vi "MAIN_STANDALONE.vi"() -> ()   [LabVIEW 2019]
uses:
  Typedefs/ESTADOS.ctl
  Typedefs/Tipo_movimiento.ctl
  Typedefs/Distancia.ctl
  Typedefs/Distancia_Z.ctl
  Typedefs/Cluster_refs_controles.ctl
  Typedefs/Cluster_tracking.ctl
  SHARED TYPES/Acciones_UI.ctl
  Typedefs/Estados_arduino.ctl
  Typedefs/Comandos.ctl
  <vilib>/Instr/_visa.llb/VISA Configure Serial Port (Instr).vi
  <vilib>/Utility/error.llb/Error Cluster From Error Code.vi
  <vilib>/ErrorRing/Error Ring.xnode
  SHARED VI'S/SHARED VI'S.lvlib
  SHARED TYPES/SHARED TYPES.lvlib
panel:
  out "?":u32
  in  "TabDepuracion":enum32{"Page 1", "Page 2"}(tab)
  in  "Tab Control":enum32{"Page 1"}(tab)
  out "Tracking_Z":i32
  in  "Distancia Z":T1=32000 items=["2cm"=64000, "1cm"=32000, "1mm"=3200, "0.5mm"=1600]
  out "Movimiento ejecutado?":bool caption="MOVIMIENTO NO EJECUTADO"
  out "Tracking_Y":i32
  out "Tracking_X":i32
  out "TRAMA DE MOVIMIENTO ENVIADA":string
  out "MENSAJES AL USUARIO":string
  in  "COMENZAR MOVIMIENTO":bool
  in  "HOME":bool
  in  "Avance":bool
  in  "Retroceso":bool
  in  "Derecha":bool
  in  "Izquierda":bool
  in  "STOP PROGRAM":bool
  in  "Sube Z":bool
  in  "Baja Z":bool
  out "ESTADO FSM":T2
  out "MOVIMIENTO SOLICITADO":T3=enum."AVANZAR"
  in  "Distancia X/Y":T4=9100 items=["60cm"=54600, "50cm"=45500, "45cm"=40950, "40cm"=36400, "35cm"=31850, "30cm"=27300, "25cm"=22750, "20cm"=18200, "15cm"=13650, "10cm"=9100, "5cm"=4550, "1cm"=910, "5mm"=455, "1mm"=91, "0.5mm"=45, "0.1mm"=9, "1 paso "=1]
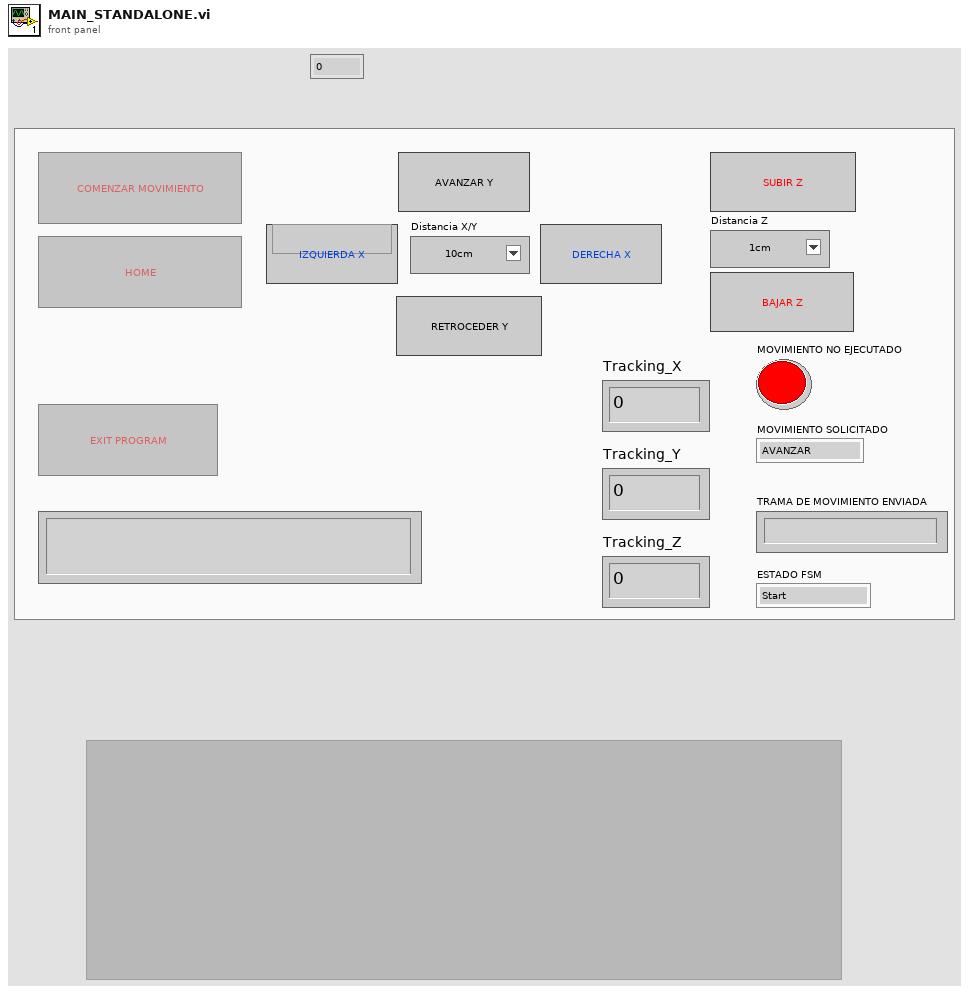
[diagram p1: front panel]
types:
  T1 = typedef "Distancia_Z.ctl" = i32
  T2 = typedef "ESTADOS.ctl" = enum16{"Start", "Ping_Arduino", "Init Refs", "Check Button", "Check Limits", "Home", "Cabezal Posicion Inicio", "Terminaste posicion inicio?", "Terminar", "Salir Arduino", "Envio Parametros Movimiento", "Recepcion Comando?", "Terminaste Movimiento?", "Adquirir Coordenada", "Terminaste Home?", "Salir"}
  T3 = typedef "Tipo_movimiento.ctl" = enum16{"NINGUNO", "AVANZAR", "RETROCEDER", "DERECHA", "IZQUIERDA", "SUBIRZ", "BAJARZ", "HOME", "HOME_Z"}
  T4 = typedef "Distancia.ctl" = i32
  T5 = typedef "Cluster_tracking.ctl" = cluster{"PasosAcumulados_Y":i32, "PasosAcumulados_X":i32, "PasosAcumulados_Z":i32, "Coord.Adquirida_X":i32, "Coord.Adquirida_Y":i32, "Coord.Adquirida_Z":i32}
  T6 = typedef "Cluster_refs_controles.ctl" = cluster{"Comenzar mov":refnum<vi>, "Home":refnum<vi>, "Izq":refnum<vi>, "Der":refnum<vi>, "Stop Program":refnum<vi>, "Avanzar":refnum<vi>, "Bajar Z":refnum<vi>, "Distancia":refnum<vi>, "Subir Z":refnum<vi>, "Retroc":refnum<vi>, "MENSAJES AL USUARIO":refnum<vi>, "Trama enviada":refnum<vi>, "Movimiento ejecutado?":refnum<vi>}
  T7 = typedef "SHARED TYPES.lvlib/Acciones_UI.ctl" = enum16{"Activar", "Desactivar", "Reiniciar default"}
  T8 = enum8{"Enabled", "Disabled", "Disabled and Grayed Out"}
  T9 = typedef "Comandos.ctl" = enum16{"H", "FH", "FI", "FX", "FY", "FZ", "I", "OK"}
  T10 = typedef "Estados_arduino.ctl" = enum16{"2", "3", "4", "5", "6", "7", "9", "8"}
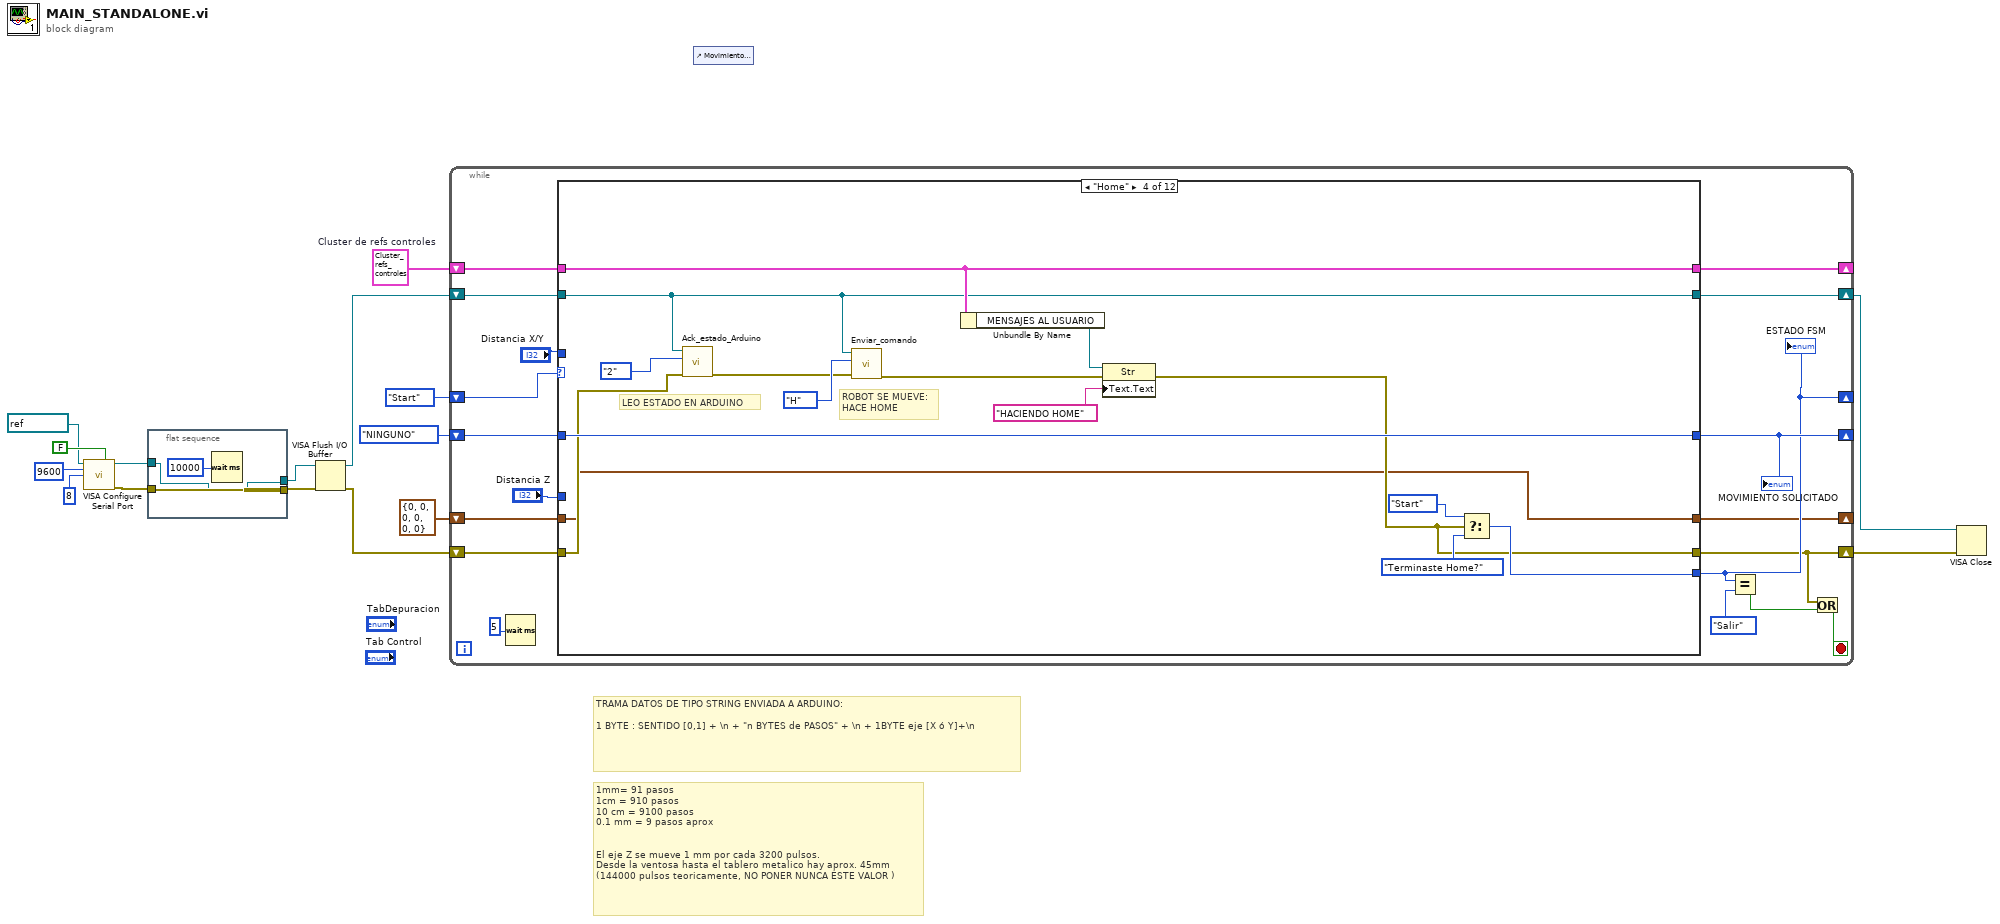
[diagram p0: block diagram]
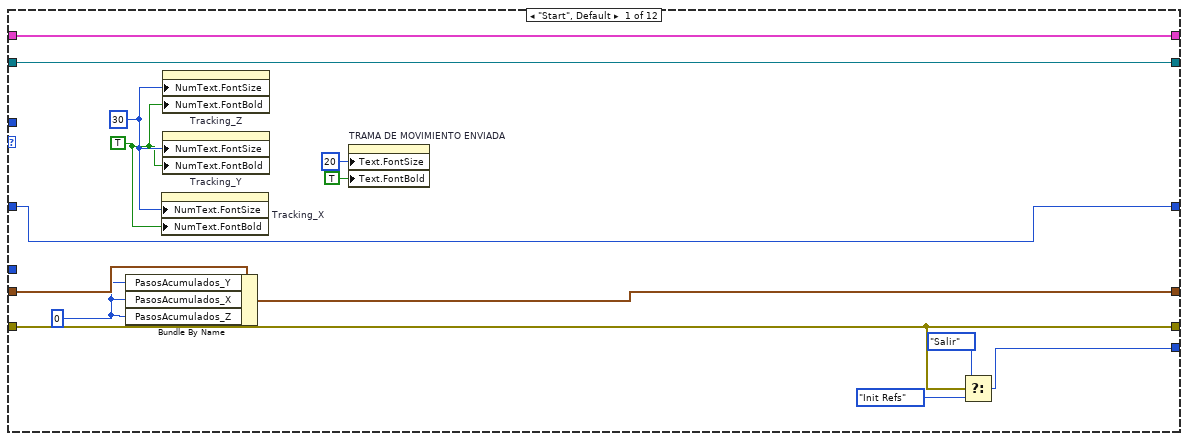
[diagram p2: hidden frame]
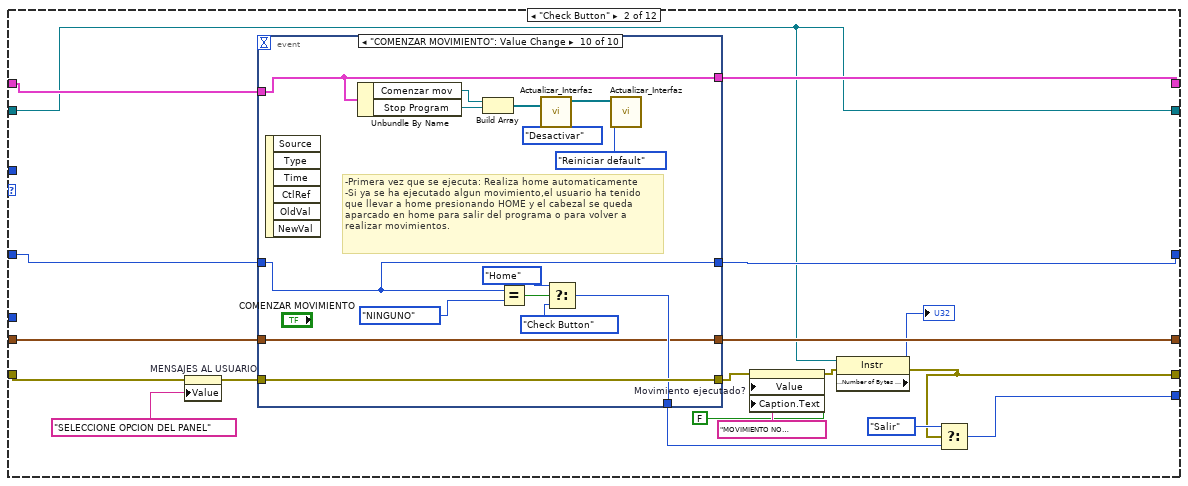
[diagram p3: hidden frame]
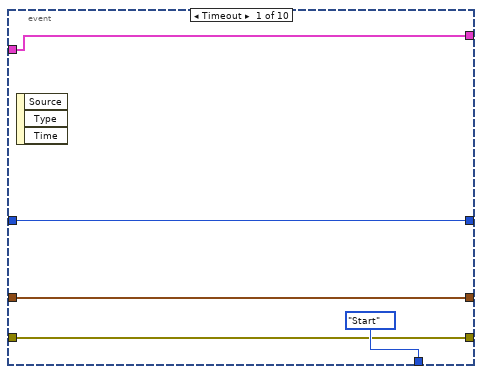
[diagram p4: hidden frame]
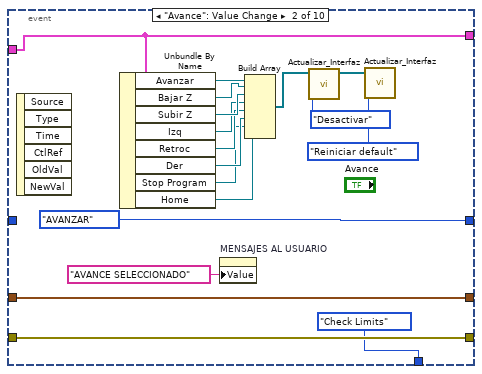
[diagram p5: hidden frame]
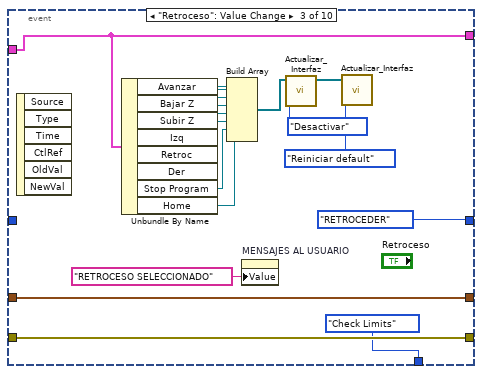
[diagram p6: hidden frame]
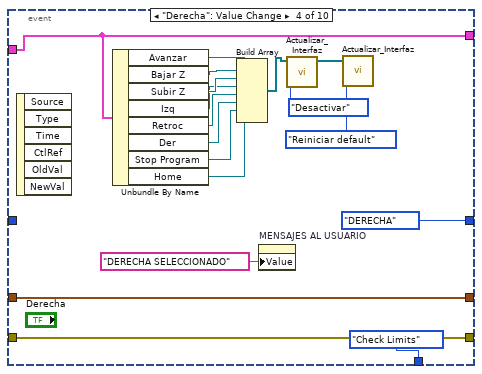
[diagram p7: hidden frame]
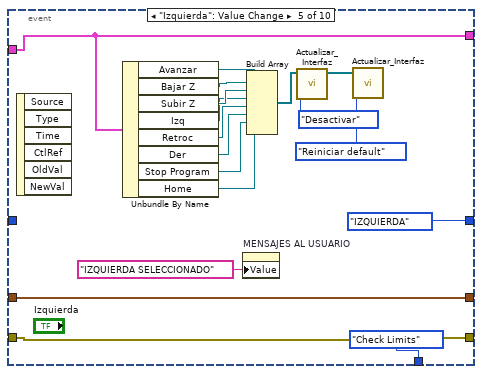
[diagram p8: hidden frame]
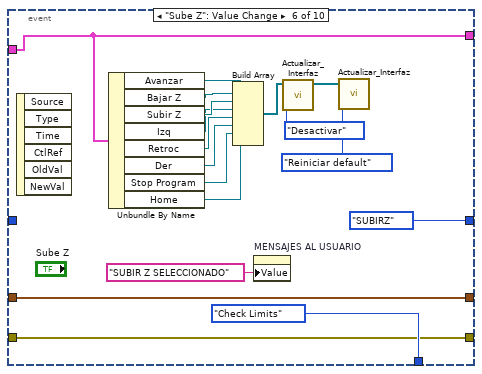
[diagram p9: hidden frame]
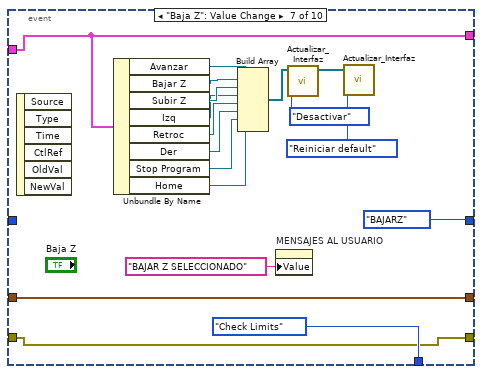
[diagram p10: hidden frame]
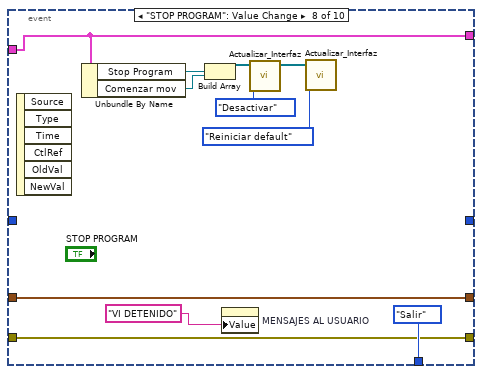
[diagram p11: hidden frame]
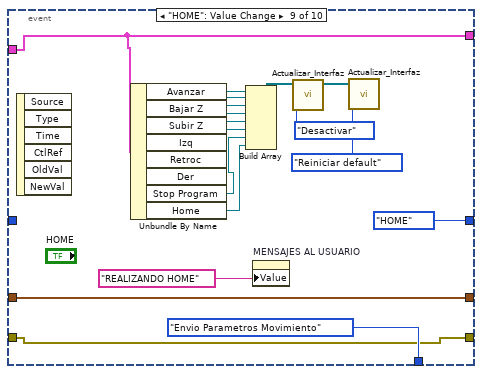
[diagram p12: hidden frame]
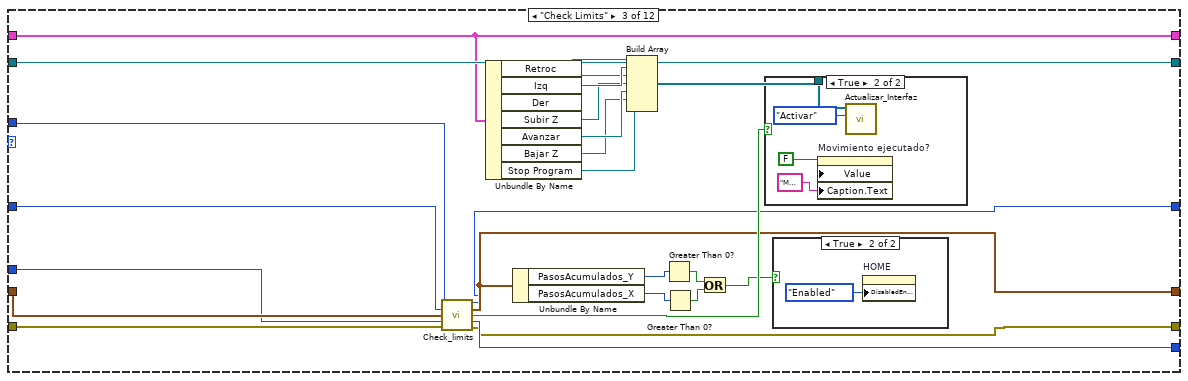
[diagram p13: hidden frame]
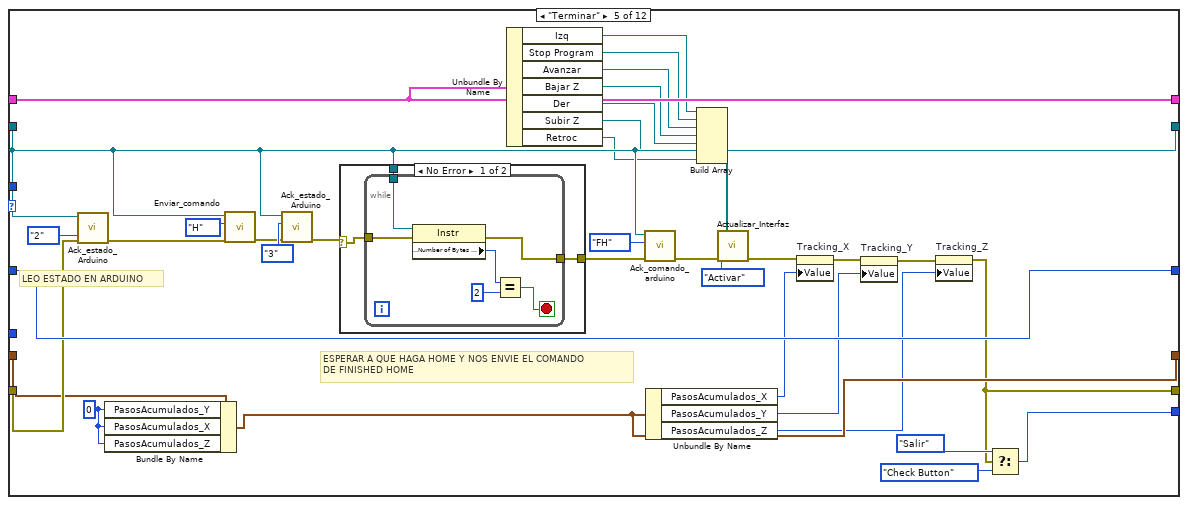
[diagram p16: hidden frame]
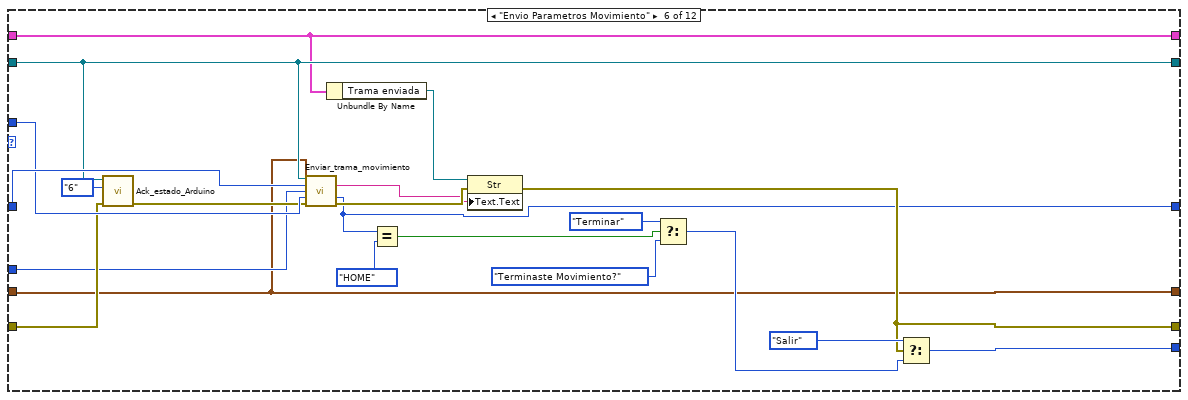
[diagram p18: hidden frame]
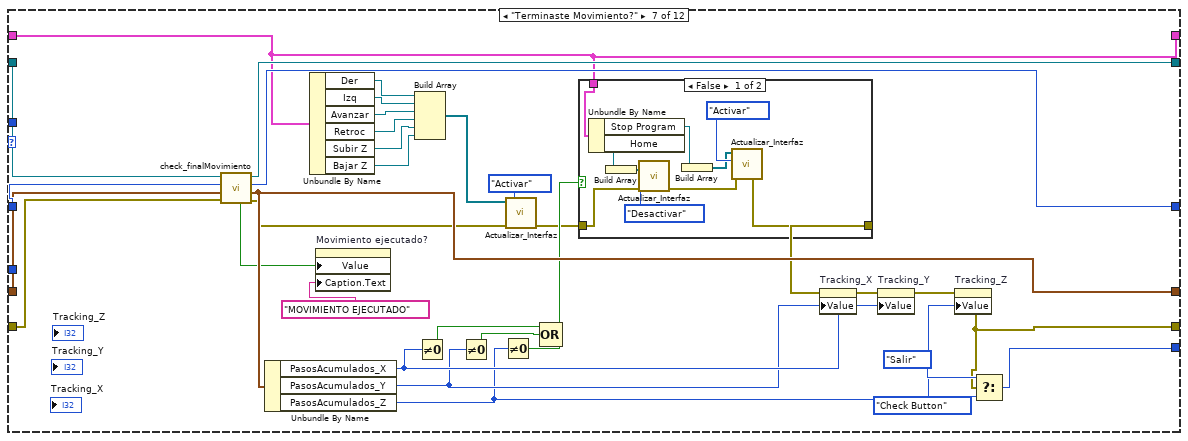
[diagram p19: hidden frame]
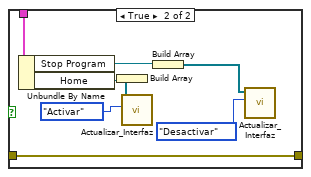
[diagram p20: hidden frame]
diagram:
  w6 = T6 {"Comenzar mov"=refnum, "Home"=refnum, "Izq"=refnum, "Der"=refnum, "Stop Program"=refnum, "Avanzar"=refnum, "Bajar Z"=refnum, "Distancia"=refnum, "Subir Z"=refnum, "Retroc"=refnum, "MENSAJES AL USUARIO"=refnum, "Trama enviada"=refnum, "Movimiento ejecutado?"=refnum}  # Cluster de refs controles
  # "1mm= 91 pasos\n1cm = 910 pasos\n10 cm = 9100 pasos\n0.1 mm = 9 pasos aprox\n\n\nEl eje Z se mueve 1 mm por cada 3200 pulsos. \nDesde la ventosa hasta el tablero metalico hay aprox. 45mm \n(144000 pulsos teoricamente, NO PONER NUNCA ÉSTE VALOR )"
  # "TRAMA DATOS DE TIPO STRING ENVIADA A ARDUINO:\n\n1 BYTE : SENTIDO [0,1] + \\n + \"n BYTES de PASOS\" + \\n + 1BYTE eje [X ó Y]+\\n"
  n1 = call-poly "VISA Configure Serial Port"("VISA resource name"=refnum<visa-resource-name> "COM4", "Enable Termination\nChar (T)"=FALSE ("Enable Termination\nChar (T)"), "baud rate (9600)"=u32 9600, "data bits (8)"=u16 8) -> ("VISA resource name out"=w5:refnum<visa-resource-name>, "error out"=w14:errorcluster)  [unwired: 10 in]
  n2 = flat-sequence {
    tunnel: [w19] -> w9
    tunnel: w14 -> [w19]
    tunnel: [w17] -> w4
    tunnel: w5 -> [w17]
    frame #0 {
      n3 = Wait (ms)(milliseconds to wait=u32 10000) -> ()  [unwired: 1 out]
    }
  }
  n4 = VISA Flush I/O Buffer(VISA resource name=w4, error in (no error)=w9) -> (VISA resource name out=w3:refnum<visa-resource-name>, error out=w2:errorcluster)  [unwired: 1 in]
  n5 = while {
    shift-right: [w25] -> w10
    shift-left: w2 -> [w34]
    shift-right: [w33] -> w11
    shift-left: w3 -> [w35]
    shift-right: [w29] -> _
    shift-left: w6 -> [w30]
    shift-right: [w27] -> _
    shift-left: ESTADOS."Start" ("Enum") -> [w36]
    shift-right: [w31] -> _
    shift-left: Tipo_movimiento."NINGUNO" ("Enum") -> [w32]
    shift-right: [w22] -> _
    shift-left: T5 {"PasosAcumulados_Y"=0, "PasosAcumulados_X"=0, "PasosAcumulados_Z"=0, "Coord.Adquirida_X"=0, "Coord.Adquirida_Y"=0, "Coord.Adquirida_Z"=0} ("Cluster_Tracking") -> [w23]
    stop <- w28 stop-if-true
    n6 = Wait (ms)(milliseconds to wait=u32 5) -> ()  [unwired: 1 out]
    n7 = case shown="\"Home\"" w36 {
      tunnel: w35 -> [w47 w52 w252 w259 w296 w335 w369 w410 w447 w465 w483 w524]
      tunnel: w34 -> [w51 w61 w250 w262 w305 w334 w368 w411 w443 w467 w484 w533]
      tunnel: [w51 w53 w231 w266 w273 w321 w351 w390 w443 w463 w482 w523] -> w25
      tunnel: [w48 w67 w249 w270 w302 w331 w365 w412 w444 w466 w486 w527] -> w27
      tunnel: [w47 w52 w252 w259 w296 w335 w370 w413 w447 w465 w483 w524] -> w33
      tunnel: w32 -> [w46 w64 w248 w271 w307 w338 w371 _ _ _ _ _]
      tunnel: "Distancia X/Y" -> [_ _ w251 _ _ w337 _ _ _ _ _ _]
      tunnel: [w46 w66 w229 w271 w307 w320 w364 _ _ _ _ _] -> w31
      tunnel: w30 -> [w42 w70 w247 w267 w293 w325 w347 w405 w461 w464 w485 w526]
      tunnel: [w42 w69 w247 w267 w293 w325 w347 w405 w448 w464 w485 w526] -> w29
      tunnel: w23 -> [w45 w63 w238 w261 w287 w318 w361 w406 w438 w462 w481 w525]
      tunnel: [w44 w62 w233 w261 w284 w318 w360 w406 w438 w462 w481 w525] -> w22
      tunnel: "Distancia Z" -> [_ _ w230 _ _ w319 _ _ _ _ _ _]
      frame "Start", Default {
        w41 = u32 30 ("Text.Font:Size")
        w40 = TRUE ("Text.Font:Bold")
        w43 = 0 ("PasosAcumulados_Y")
        n8 = Bundle By Name(cluster=w45, "PasosAcumulados_Y"=w43, "PasosAcumulados_X"=w43, "PasosAcumulados_Z"=w43) -> (w44:T5)
        n9 = property on="Tracking_X" class="DigNum (strict)"("NumText.FontSize"=w41, "NumText.FontBold"=w40) -> ()  [unwired: 2 in, 2 out]
        n10 = property on="Tracking_Z" class="DigNum (strict)"("NumText.FontSize"=w41, "NumText.FontBold"=w40) -> ()  [unwired: 2 in, 2 out]
        n11 = property on="Tracking_Y" class="DigNum (strict)"("NumText.FontSize"=w41, "NumText.FontBold"=w40) -> ()  [unwired: 2 in, 2 out]
        n12 = property on="TRAMA DE MOVIMIENTO ENVIADA" class="Str"("Text.FontSize"=u32 20 ("Text.Font:Size"), "Text.FontBold"=TRUE ("Text.Font:Bold")) -> ()  [unwired: 2 in, 2 out]
        n13 = Select(t=ESTADOS."Salir", s=w51, f=ESTADOS."Init Refs" ("Enum")) -> (s? t:f=w48:T2)
      }
      frame "Check Button" {
        n14 = property on="MENSAJES AL USUARIO" class="Str"(error in=w61, "Value"="SELECCIONE OPCION DEL PANEL" ("MENSAJES AL USUARIO")) -> (error out=w60:errorcluster)  [unwired: 1 in, 1 out]
        n15 = event shown="[9] \"COMENZAR MOVIMIENTO\": Value Change" {
          selector: _ -> [_ _ _ _ _ _ _ _ _ _]
          dyn-events: _ -> [_ _ _ _ _ _ _ _ _ _]
          timeout: _ -> [_ _ _ _ _ _ _ _ _ _]
          tunnel: w70 -> [w75 w93 w102 w120 w136 w152 w170 w189 w199 w224]
          tunnel: [w75 w93 w102 w120 w136 w152 w170 w189 w199 w224] -> w69
          tunnel: [w74 Tipo_movimiento."AVANZAR" Tipo_movimiento."RETROCEDER" Tipo_movimiento."DERECHA" Tipo_movimiento."IZQUIERDA" Tipo_movimiento."SUBIRZ" Tipo_movimiento."BAJARZ" _ Tipo_movimiento."HOME" w216] -> w66
          tunnel: [ESTADOS."Start" ESTADOS."Check Limits" ("f") ESTADOS."Check Limits" ("f") ESTADOS."Check Limits" ("f") ESTADOS."Check Limits" ("f") ESTADOS."Check Limits" ("Enum") ESTADOS."Check Limits" ("Enum") ESTADOS."Salir" ("Enum") ESTADOS."Envio Parametros Movimiento" w215] -> w65
          tunnel: [w72 w79 w96 w114 w132 w163 w181 w187 w211 w221] -> w56
          tunnel: w60 -> [w72 w79 w96 w114 w132 w163 w181 w187 w211 w221]
          tunnel: w64 -> [w74 _ _ _ _ _ _ _ _ w216]
          tunnel: w63 -> [w71 w78 w97 w115 w133 w149 w167 w186 w196 w213]
          tunnel: [w71 w78 w97 w115 w133 w149 w167 w186 w196 w213] -> w62
          event Timeout {
            n16 = event-data() -> ()  [unwired: 1 in, 3 out]
          }
          event "Avance": Value Change {
            n17 = event-data() -> ()  [unwired: 1 in, 6 out]
            n18 = Unbundle By Name(w93) -> ("Avanzar"=w92:refnum<vi>, "Bajar Z"=w87:refnum<vi>, "Subir Z"=w86:refnum<vi>, "Izq"=w85:refnum<vi>, "Retroc"=w84:refnum<vi>, "Der"=w83:refnum<vi>, "Stop Program"=w82:refnum<vi>, "Home"=w81:refnum<vi>)
            n19 = property on="MENSAJES AL USUARIO" class="Str"("Value"="AVANCE SELECCIONADO" ("MENSAJES AL USUARIO")) -> ()  [unwired: 2 in, 2 out]
            n20 = Build Array(w92, w87, w86, w85, w84, w83, w82, w81) -> (w91:refnum<vi>[])
            n21 = call "Actualizar_Interfaz.vi"("Enum"=Acciones_UI."Desactivar", "Controls"=w91) -> ("Controls 2"=w89:refnum<vi>[])  [unwired: 8 in, 1 out]
            n22 = call "Actualizar_Interfaz.vi"("Enum"=Acciones_UI."Reiniciar default", "Controls"=w89) -> ()  [unwired: 8 in, 2 out]
          }
          event "Retroceso": Value Change {
            n23 = event-data() -> ()  [unwired: 1 in, 6 out]
            n24 = Unbundle By Name(w102) -> ("Avanzar"=w111:refnum<vi>, "Bajar Z"=w107:refnum<vi>, "Subir Z"=w106:refnum<vi>, "Izq"=w105:refnum<vi>, "Retroc"=w104:refnum<vi>, "Der"=w103:refnum<vi>, "Stop Program"=w100:refnum<vi>, "Home"=w99:refnum<vi>)
            n25 = Build Array(w111, w107, w106, w105, w104, w103, w100, w99) -> (w101:refnum<vi>[])
            n26 = property on="MENSAJES AL USUARIO" class="Str"("Value"="RETROCESO SELECCIONADO" ("MENSAJES AL USUARIO")) -> ()  [unwired: 2 in, 2 out]
            n27 = call "Actualizar_Interfaz.vi"("Enum"=Acciones_UI."Desactivar", "Controls"=w101) -> ("Controls 2"=w109:refnum<vi>[])  [unwired: 8 in, 1 out]
            n28 = call "Actualizar_Interfaz.vi"("Enum"=Acciones_UI."Reiniciar default", "Controls"=w109) -> ()  [unwired: 8 in, 2 out]
          }
          event "Derecha": Value Change {
            n29 = event-data() -> ()  [unwired: 1 in, 6 out]
            n30 = Unbundle By Name(w120) -> ("Avanzar"=w129:refnum<vi>, "Bajar Z"=w125:refnum<vi>, "Subir Z"=w124:refnum<vi>, "Izq"=w123:refnum<vi>, "Retroc"=w122:refnum<vi>, "Der"=w121:refnum<vi>, "Stop Program"=w119:refnum<vi>, "Home"=w117:refnum<vi>)
            n31 = Build Array(w129, w125, w124, w123, w122, w121, w119, w117) -> (w118:refnum<vi>[])
            n32 = property on="MENSAJES AL USUARIO" class="Str"("Value"="DERECHA SELECCIONADO" ("MENSAJES AL USUARIO")) -> ()  [unwired: 2 in, 2 out]
            n33 = call "Actualizar_Interfaz.vi"("Enum"=Acciones_UI."Desactivar", "Controls"=w118) -> ("Controls 2"=w127:refnum<vi>[])  [unwired: 8 in, 1 out]
            n34 = call "Actualizar_Interfaz.vi"("Enum"=Acciones_UI."Reiniciar default", "Controls"=w127) -> ()  [unwired: 8 in, 2 out]
          }
          event "Izquierda": Value Change {
            n35 = event-data() -> ()  [unwired: 1 in, 6 out]
            n36 = Unbundle By Name(w136) -> ("Avanzar"=w147:refnum<vi>, "Bajar Z"=w143:refnum<vi>, "Subir Z"=w142:refnum<vi>, "Izq"=w141:refnum<vi>, "Retroc"=w140:refnum<vi>, "Der"=w139:refnum<vi>, "Stop Program"=w138:refnum<vi>, "Home"=w135:refnum<vi>)
            n37 = property on="MENSAJES AL USUARIO" class="Str"("Value"="IZQUIERDA SELECCIONADO" ("MENSAJES AL USUARIO")) -> ()  [unwired: 2 in, 2 out]
            n38 = Build Array(w147, w143, w142, w141, w140, w139, w138, w135) -> (w137:refnum<vi>[])
            n39 = call "Actualizar_Interfaz.vi"("Enum"=Acciones_UI."Desactivar", "Controls"=w137) -> ("Controls 2"=w145:refnum<vi>[])  [unwired: 8 in, 1 out]
            n40 = call "Actualizar_Interfaz.vi"("Enum"=Acciones_UI."Reiniciar default", "Controls"=w145) -> ()  [unwired: 8 in, 2 out]
          }
          event "Sube Z": Value Change {
            n41 = event-data() -> ()  [unwired: 1 in, 6 out]
            n42 = Unbundle By Name(w152) -> ("Avanzar"=w162:refnum<vi>, "Bajar Z"=w158:refnum<vi>, "Subir Z"=w157:refnum<vi>, "Izq"=w156:refnum<vi>, "Retroc"=w155:refnum<vi>, "Der"=w154:refnum<vi>, "Stop Program"=w153:refnum<vi>, "Home"=w150:refnum<vi>)
            n43 = Build Array(w162, w158, w157, w156, w155, w154, w153, w150) -> (w151:refnum<vi>[])
            n44 = property on="MENSAJES AL USUARIO" class="Str"("Value"="SUBIR Z SELECCIONADO" ("MENSAJES AL USUARIO")) -> ()  [unwired: 2 in, 2 out]
            n45 = call "Actualizar_Interfaz.vi"("Enum"=Acciones_UI."Desactivar", "Controls"=w151) -> ("Controls 2"=w160:refnum<vi>[])  [unwired: 8 in, 1 out]
            n46 = call "Actualizar_Interfaz.vi"("Enum"=Acciones_UI."Reiniciar default", "Controls"=w160) -> ()  [unwired: 8 in, 2 out]
          }
          event "Baja Z": Value Change {
            n47 = event-data() -> ()  [unwired: 1 in, 6 out]
            n48 = Unbundle By Name(w170) -> ("Avanzar"=w180:refnum<vi>, "Bajar Z"=w176:refnum<vi>, "Subir Z"=w175:refnum<vi>, "Izq"=w174:refnum<vi>, "Retroc"=w173:refnum<vi>, "Der"=w172:refnum<vi>, "Stop Program"=w171:refnum<vi>, "Home"=w168:refnum<vi>)
            n49 = Build Array(w180, w176, w175, w174, w173, w172, w171, w168) -> (w169:refnum<vi>[])
            n50 = property on="MENSAJES AL USUARIO" class="Str"("Value"="BAJAR Z SELECCIONADO" ("MENSAJES AL USUARIO")) -> ()  [unwired: 2 in, 2 out]
            n51 = call "Actualizar_Interfaz.vi"("Enum"=Acciones_UI."Desactivar", "Controls"=w169) -> ("Controls 2"=w178:refnum<vi>[])  [unwired: 8 in, 1 out]
            n52 = call "Actualizar_Interfaz.vi"("Enum"=Acciones_UI."Reiniciar default", "Controls"=w178) -> ()  [unwired: 8 in, 2 out]
          }
          event "STOP PROGRAM": Value Change {
            n53 = event-data() -> ()  [unwired: 1 in, 6 out]
            n54 = Unbundle By Name(w189) -> ("Stop Program"=w194:refnum<vi>, "Comenzar mov"=w185:refnum<vi>)
            n55 = Build Array(w194, w185) -> (w193:refnum<vi>[])
            n56 = property on="MENSAJES AL USUARIO" class="Str"("Value"="VI DETENIDO" ("MENSAJES AL USUARIO")) -> ()  [unwired: 2 in, 2 out]
            n57 = call "Actualizar_Interfaz.vi"("Enum"=Acciones_UI."Desactivar", "Controls"=w193) -> ("Controls 2"=w191:refnum<vi>[])  [unwired: 8 in, 1 out]
            n58 = call "Actualizar_Interfaz.vi"("Enum"=Acciones_UI."Reiniciar default", "Controls"=w191) -> ()  [unwired: 8 in, 2 out]
          }
          event "HOME": Value Change {
            n59 = event-data() -> ()  [unwired: 1 in, 6 out]
            n60 = Unbundle By Name(w199) -> ("Avanzar"=w209:refnum<vi>, "Bajar Z"=w204:refnum<vi>, "Subir Z"=w203:refnum<vi>, "Izq"=w202:refnum<vi>, "Retroc"=w201:refnum<vi>, "Der"=w200:refnum<vi>, "Stop Program"=w198:refnum<vi>, "Home"=w197:refnum<vi>)
            n61 = Build Array(w209, w204, w203, w202, w201, w200, w198, w197) -> (w208:refnum<vi>[])
            n62 = property on="MENSAJES AL USUARIO" class="Str"("Value"="REALIZANDO HOME" ("MENSAJES AL USUARIO")) -> ()  [unwired: 2 in, 2 out]
            n63 = call "Actualizar_Interfaz.vi"("Enum"=Acciones_UI."Desactivar", "Controls"=w208) -> ("Controls 2"=w206:refnum<vi>[])  [unwired: 8 in, 1 out]
            n64 = call "Actualizar_Interfaz.vi"("Enum"=Acciones_UI."Reiniciar default", "Controls"=w206) -> ()  [unwired: 8 in, 2 out]
          }
          event "COMENZAR MOVIMIENTO": Value Change {
            # "-Primera vez que se ejecuta: Realiza home automaticamente\n-Si ya se ha ejecutado algun movimiento,el usuario ha tenido que llevar a home presionando HOME y el cabezal se queda aparcado en home para salir del programa o para volver a realizar movimientos."
            n65 = event-data() -> ()  [unwired: 1 in, 6 out]
            n66 = Unbundle By Name(w224) -> ("Comenzar mov"=w227:refnum<vi>, "Stop Program"=w214:refnum<vi>)
            n67 = Build Array(w227, w214) -> (w226:refnum<vi>[])
            n68 = Equal?(x=w216, y=Tipo_movimiento."NINGUNO") -> (x = y?=w219:bool)
            n69 = call "Actualizar_Interfaz.vi"("Enum"=Acciones_UI."Desactivar", "Controls"=w226) -> ("Controls 2"=w223:refnum<vi>[])  [unwired: 8 in, 1 out]
            n70 = Select(t=ESTADOS."Home", s=w219, f=ESTADOS."Check Button") -> (s? t:f=w215:T2)
            n71 = call "Actualizar_Interfaz.vi"("Enum"=Acciones_UI."Reiniciar default", "Controls"=w223) -> ()  [unwired: 8 in, 2 out]
          }
        }
        n72 = property on="Movimiento ejecutado?" class="Bool (strict)"(error in=w56, "Value"=FALSE ("Movimiento ejecutado?"), "Caption.Text"="MOVIMIENTO NO EJECUTADO" ("Label.Text")) -> (error out=w54:errorcluster)  [unwired: 1 in, 1 out]
        n73 = property class="Instr"(reference=w52, error in=w54) -> (error out=w53:errorcluster, "Serial Settings:Number of Bytes at Serial Port"=→"?":u32)  [unwired: 1 out]
        n74 = Select(t=ESTADOS."Salir", s=w53, f=w65) -> (s? t:f=w67:T2)
      }
      frame "Check Limits" {
        n75 = call "Check_limits.vi"("Distancia X/Y"=w251, "Tipo Movimiento"=w248, "Cluster_Tracking"=w238, "Distancia Z"=w230, "error in (no error)"=w250) -> ("Tipo Movimiento 2"=w229:T3, "Cluster_Tracking 2"=w233:T5, "Limite sobrepasado?"=w246:bool, "Estado"=w249:T2, "error out"=w231:errorcluster)  [unwired: 6 in]
        n76 = Unbundle By Name(w247) -> ("Retroc"=w245:refnum<vi>, "Izq"=w244:refnum<vi>, "Der"=w243:refnum<vi>, "Subir Z"=w242:refnum<vi>, "Avanzar"=w241:refnum<vi>, "Bajar Z"=w240:refnum<vi>, "Stop Program"=w228:refnum<vi>)
        n77 = Unbundle By Name(w233) -> ("PasosAcumulados_Y"=w236:i32, "PasosAcumulados_X"=w235:i32)
        n78 = Build Array(w245, w244, w243, w242, w241, w240, w228) -> (w239:refnum<vi>[])
        n79 = Greater Than 0?(x=w236) -> (x > 0?=w237:bool)
        n80 = Greater Than 0?(x=w235) -> (x > 0?=w234:bool)
        n81 = Or(x=w237, y=w234) -> (x .or. y?=w232:bool)
        n82 = case shown="True" w246 {
          tunnel: w239 -> [_ w257]
          frame False {
          }
          frame True {
            n83 = property on="Movimiento ejecutado?" class="Bool (strict)"("Value"=FALSE ("Movimiento ejecutado"), "Caption.Text"="MOVIMIENTO NO EJECUTADO" ("Label.Text")) -> ()  [unwired: 2 in, 2 out]
            n84 = call "Actualizar_Interfaz.vi"("Enum"=Acciones_UI."Activar", "Controls"=w257) -> ()  [unwired: 8 in, 2 out]
          }
        }
        n85 = case shown="True" w232 {
          frame False {
          }
          frame True {
            n86 = property on="HOME" class="Bool"("DisabledEnum"=T8."Enabled" ("Disabled")) -> ()  [unwired: 2 in, 2 out]
          }
        }
      }
      frame "Home" {
        # "ROBOT SE MUEVE:\nHACE HOME"
        # "LEO ESTADO EN ARDUINO"
        n87 = call "Ack_estado_Arduino.vi"("error in (no error)"=w262, "Enum"=Estados_arduino."2", "VISA resource name"=w259) -> ("error out"=w258:errorcluster)  [unwired: 6 in, 2 out]
        n88 = call "Enviar_comando.vi"("error in (no error)"=w258, "Enum"=Comandos."H", "VISA resource name"=w259) -> ("error out"=w265:errorcluster)  [unwired: 6 in, 2 out]
        n89 = Unbundle By Name(w267) -> ("MENSAJES AL USUARIO"=w264:refnum<vi>)
        n90 = property class="Str"(reference=w264, error in=w265, "Text.Text"="HACIENDO HOME") -> (error out=w266:errorcluster)  [unwired: 1 out]
        n91 = Select(t=ESTADOS."Start" ("Enum"), s=w266, f=ESTADOS."Terminaste Home?" ("Enum")) -> (s? t:f=w270:T2)
      }
      frame "Terminar" {
        w276 = 0 ("PasosAcumulados_Y")
        # "LEO ESTADO EN ARDUINO"
        # "ESPERAR A QUE HAGA HOME Y NOS ENVIE EL COMANDO\nDE FINISHED HOME"
        n92 = call "Ack_estado_Arduino.vi"("error in (no error)"=w305, "Enum"=Estados_arduino."2", "VISA resource name"=w296) -> ("error out"=w301:errorcluster)  [unwired: 6 in, 2 out]
        n93 = Bundle By Name(cluster=w287, "PasosAcumulados_Y"=w276, "PasosAcumulados_X"=w276, "PasosAcumulados_Z"=w276) -> (w284:T5)
        n94 = call "Enviar_comando.vi"("error in (no error)"=w301, "Enum"=Comandos."H", "VISA resource name"=w296) -> ("error out"=w295:errorcluster)  [unwired: 6 in, 2 out]
        n95 = call "Ack_estado_Arduino.vi"("error in (no error)"=w295, "Enum"=Estados_arduino."3", "VISA resource name"=w296) -> ("error out"=w297:errorcluster)  [unwired: 6 in, 2 out]
        n96 = case shown="No Error" w297 {
          selector: w297 -> [w308 w317]
          tunnel: [w310 w317] -> w299
          tunnel: w296 -> [w309 _]
          frame No Error {
            n97 = while {
              tunnel: [w316] -> w310
              tunnel: w309 -> [w312]
              tunnel: w308 -> [w311]
              stop <- w313 stop-if-true
              n98 = property class="Instr"(reference=w312, error in=w311) -> (error out=w316:errorcluster, "Serial Settings:Number of Bytes at Serial Port"=w315:u32)  [unwired: 1 out]
              n99 = Equal?(x=w315, y=u32 2) -> (x = y?=w313:bool)
            }
          }
          frame Error {
          }
        }
        n100 = Unbundle By Name(w293) -> ("Izq"=w292:refnum<vi>, "Stop Program"=w288:refnum<vi>, "Avanzar"=w281:refnum<vi>, "Bajar Z"=w280:refnum<vi>, "Der"=w279:refnum<vi>, "Subir Z"=w278:refnum<vi>, "Retroc"=w277:refnum<vi>)
        n101 = call "Ack_comando_arduino.vi"("error in (no error)"=w299, 10:Comandos."FH", "VISA resource name"=w296) -> ("error IO"=w291:errorcluster)  [unwired: 6 in, 2 out]
        n102 = Unbundle By Name(w284) -> ("PasosAcumulados_X"=w283:i32, "PasosAcumulados_Y"=w282:i32, "PasosAcumulados_Z"=w274:i32)
        n103 = Build Array(w292, w288, w281, w280, w279, w278, w277) -> (w290:refnum<vi>[])
        n104 = call "Actualizar_Interfaz.vi"("error in (no error)"=w291, "Enum"=Acciones_UI."Activar", "Controls"=w290) -> ("error out"=w286:errorcluster)  [unwired: 7 in, 1 out]
        n105 = property on="Tracking_X" class="DigNum (strict)"(error in=w286, "Value"=w283) -> (error out=w285:errorcluster)  [unwired: 1 in, 1 out]
        n106 = property on="Tracking_Y" class="DigNum (strict)"(error in=w285, "Value"=w282) -> (error out=w275:errorcluster)  [unwired: 1 in, 1 out]
        n107 = property on="Tracking_Z" class="DigNum (strict)"(error in=w275, "Value"=w274) -> (error out=w273:errorcluster)  [unwired: 1 in, 1 out]
        n108 = Select(t=ESTADOS."Salir" ("Enum"), s=w273, f=ESTADOS."Check Button") -> (s? t:f=w302:T2)
      }
      frame "Envio Parametros Movimiento" {
        n109 = call "Ack_estado_Arduino.vi"("error in (no error)"=w334, "Enum"=Estados_arduino."6", "VISA resource name"=w335) -> ("error out"=w333:errorcluster)  [unwired: 6 in, 2 out]
        n110 = call "Enviar_trama_movimiento.vi"("VISA resource name"=w335, "Cluster_Tracking"=w318, "Tipo movimiento"=w338, "Distancia Z"=w319, "Distancia X/Y"=w337, "error in (no error)"=w333) -> ("TRAMA ENVIADA"=w323:string, "Tipo movimiento"=w320:T3, "error out"=w324:errorcluster)  [unwired: 6 in, 1 out]
        n111 = Unbundle By Name(w325) -> ("Trama enviada"=w322:refnum<vi>)
        n112 = Equal?(x=w320, y=Tipo_movimiento."HOME") -> (x = y?=w329:bool)
        n113 = property class="Str"(reference=w322, error in=w324, "Text.Text"=w323) -> (error out=w321:errorcluster)  [unwired: 1 out]
        n114 = Select(t=ESTADOS."Terminar", s=w329, f=ESTADOS."Terminaste Movimiento?") -> (s? t:f=w326:T2)
        n115 = Select(t=ESTADOS."Salir" ("Enum"), s=w321, f=w326) -> (s? t:f=w331:T2)
      }
      frame "Terminaste Movimiento?" {
        n116 = call "check_finalMovimiento.vi"("error in (no error)"=w368, "Cluster_Tracking in"=w361, "Enum in"=w371, "VISA Refnum in"=w369) -> ("error out"=w352:errorcluster, "Cluster_Tracking out"=w360:T5, "Enum out"=w364:T3, "VISA Refnum out"=w370:refnum<visa-resource-name>, "Movimiento realizado?"=w348:bool)  [unwired: 3 in]
        n117 = Unbundle By Name(w360) -> ("PasosAcumulados_X"=w359:i32, "PasosAcumulados_Y"=w358:i32, "PasosAcumulados_Z"=w353:i32)
        n118 = Unbundle By Name(w347) -> ("Der"=w346:refnum<vi>, "Izq"=w345:refnum<vi>, "Avanzar"=w344:refnum<vi>, "Retroc"=w343:refnum<vi>, "Subir Z"=w342:refnum<vi>, "Bajar Z"=w341:refnum<vi>)
        n119 = property on="Movimiento ejecutado?" class="Bool (strict)"("Value"=w348, "Caption.Text"="MOVIMIENTO EJECUTADO" ("Label.Text")) -> ()  [unwired: 2 in, 2 out]
        n120 = Build Array(w346, w345, w344, w343, w342, w341) -> (w340:refnum<vi>[])
        n121 = Not Equal To 0?(x=w359) -> (x != 0?=w357:bool)
        n122 = Not Equal To 0?(x=w358) -> (x != 0?=w356:bool)
        n123 = Not Equal To 0?(x=w353) -> (x != 0?=w355:bool)
        n124 = call "Actualizar_Interfaz.vi"("Enum"=Acciones_UI."Activar", "Controls"=w340) -> ()  [unwired: 8 in, 2 out]
        n125 = Compound Arithmetic op=OR(w357, w356, w355) -> (w354:bool)
        n126 = case shown="False" w354 {
          tunnel: w352 -> [w376 w386]
          tunnel: [w374 w386] -> w350
          tunnel: w347 -> [w373 w385]
          frame False {
            n127 = Unbundle By Name(w373) -> ("Stop Program"=w377:refnum<vi>, "Home"=w381:refnum<vi>)
            n128 = Build Array(w381) -> (w380:refnum<vi>[])
            n129 = call "Actualizar_Interfaz.vi"("error in (no error)"=w376, "Enum"=Acciones_UI."Desactivar", "Controls"=w380) -> ("error out"=w375:errorcluster)  [unwired: 7 in, 1 out]
            n130 = Build Array(w377) -> (w372:refnum<vi>[])
            n131 = call "Actualizar_Interfaz.vi"("error in (no error)"=w375, "Enum"=Acciones_UI."Activar", "Controls"=w372) -> ("error out"=w374:errorcluster)  [unwired: 7 in, 1 out]
          }
          frame True {
            n132 = Unbundle By Name(w385) -> ("Stop Program"=w384:refnum<vi>, "Home"=w389:refnum<vi>)
            n133 = Build Array(w389) -> (w387:refnum<vi>[])
            n134 = call "Actualizar_Interfaz.vi"("Enum"=Acciones_UI."Activar", "Controls"=w387) -> ()  [unwired: 8 in, 2 out]
            n135 = Build Array(w384) -> (w382:refnum<vi>[])
            n136 = call "Actualizar_Interfaz.vi"("Enum"=Acciones_UI."Desactivar", "Controls"=w382) -> ()  [unwired: 8 in, 2 out]
          }
        }
        n137 = property on="Tracking_X" class="DigNum (strict)"(error in=w350, "Value"=w359) -> (error out=w363:errorcluster)  [unwired: 1 in, 1 out]
        n138 = property on="Tracking_Y" class="DigNum (strict)"(error in=w363, "Value"=w358) -> (error out=w362:errorcluster)  [unwired: 1 in, 1 out]
        n139 = property on="Tracking_Z" class="DigNum (strict)"(error in=w362, "Value"=w353) -> (error out=w351:errorcluster)  [unwired: 1 in, 1 out]
        n140 = Select(t=ESTADOS."Salir" ("Enum"), s=w351, f=ESTADOS."Check Button") -> (s? t:f=w365:T2)
      }
      frame "Terminaste Home?" {
        # "LEO ESTADO EN ARDUINO"
        # "ESPERAR A QUE HAGA HOME Y NOS ENVIE EL COMANDO\nDE FINISHED HOME \"FH\""
        n141 = call "Ack_estado_Arduino.vi"("error in (no error)"=w411, "Enum"=Estados_arduino."3", "VISA resource name"=w410) -> ("error out"=w407:errorcluster, "VISA resource name out"=w408:refnum<visa-resource-name>)  [unwired: 6 in, 1 out]
        n142 = case shown="No Error" w407 {
          selector: w407 -> [w419 w430]
          tunnel: [w422 w430] -> w415
          tunnel: [w421 w431] -> w414
          tunnel: w408 -> [w420 w431]
          frame No Error {
            n143 = while {
              tunnel: [w429] -> w422
              tunnel: w420 -> [w426]
              tunnel: [w424] -> w421
              tunnel: w419 -> [w425]
              stop <- w427 stop-if-true
              n144 = property class="Instr"(reference=w426, error in=w425) -> (reference out=w424:refnum<visa-resource-name>, error out=w429:errorcluster, "Serial Settings:Number of Bytes at Serial Port"=w423:u32)
              n145 = Equal?(x=w423, y=u32 2) -> (x = y?=w427:bool)
            }
          }
          frame Error {
          }
        }
        n146 = Unbundle By Name(w405) -> ("Retroc"=w402:refnum<vi>, "Izq"=w401:refnum<vi>, "Der"=w400:refnum<vi>, "Subir Z"=w399:refnum<vi>, "Avanzar"=w398:refnum<vi>, "Bajar Z"=w397:refnum<vi>, "Distancia"=w396:refnum<vi>, "Stop Program"=w395:refnum<vi>, "Movimiento ejecutado?"=w393:refnum<vi>)
        n147 = call "Ack_comando_arduino.vi"("error in (no error)"=w415, 10:Comandos."FH", "VISA resource name"=w414) -> ("error IO"=w404:errorcluster, "VISA resource name 2"=w413:refnum<visa-resource-name>)  [unwired: 6 in, 1 out]
        n148 = Build Array(w402, w401, w400, w399, w398, w397, w396, w395, w393) -> (w394:refnum<vi>[])
        n149 = call "Actualizar_Interfaz.vi"("error in (no error)"=w404, "Enum"=Acciones_UI."Activar", "Controls"=w394) -> ("error out"=w392:errorcluster)  [unwired: 7 in, 1 out]
        n150 = property on="Distancia Z" class="Ring (strict)"(error in=w392, "DisabledEnum"=T8."Enabled" ("Disabled")) -> (error out=w390:errorcluster)  [unwired: 1 in, 1 out]
        n151 = Select(t=ESTADOS."Salir" ("Enum"), s=w390, f=ESTADOS."Check Button") -> (s? t:f=w412:T2)
      }
      frame "Init Refs" {
        n152 = control-ref of="Izquierda"() -> (w457:refnum<vi>)
        n153 = control-ref of="HOME"() -> (w458:refnum<vi>)
        n154 = control-ref of="Derecha"() -> (w456:refnum<vi>)
        n155 = control-ref of="STOP PROGRAM"() -> (w455:refnum<vi>)
        n156 = control-ref of="Avance"() -> (w454:refnum<vi>)
        n157 = control-ref of="COMENZAR MOVIMIENTO"() -> (w442:refnum<vi>)
        n158 = control-ref of="Baja Z"() -> (w453:refnum<vi>)
        n159 = control-ref of="Distancia xy"() -> (w437:refnum<vi>)
        n160 = control-ref of="Sube Z"() -> (w452:refnum<vi>)
        n161 = control-ref of="Retroceso"() -> (w451:refnum<vi>)
        n162 = control-ref of="Movimiento ejecutado?"() -> (w436:refnum<vi>)
        n163 = control-ref of="MENSAJES AL USUARIO"() -> (w434:refnum<vi>)
        n164 = control-ref of="TRAMA DE MOVIMIENTO ENVIADA"() -> (w439:refnum<vi>)
        n165 = property class="Str"(reference=w434, "Text.FontSize"=u32 30 ("Text.Font:Size"), "Text.FontBold"=TRUE ("Text.Font:Bold")) -> ()  [unwired: 1 in, 2 out]
        n166 = Bundle By Name(cluster=w461, "Comenzar mov"=w442, "Home"=w458, "Izq"=w457, "Der"=w456, "Stop Program"=w455, "Avanzar"=w454, "Bajar Z"=w453, "Distancia"=w437, "Subir Z"=w452, "Retroc"=w451, "MENSAJES AL USUARIO"=w434, "Trama enviada"=w439, "Movimiento ejecutado?"=w436) -> (w448:T6)
        n167 = property on="Distancia Z" class="Ring (strict)"("DisabledEnum"=T8."Disabled and Grayed Out" ("Disabled")) -> ()  [unwired: 2 in, 2 out]
        n168 = Build Array(w458, w457, w456, w455, w454, w453, w437, w452, w451, w442, w436) -> (w450:refnum<vi>[])
        n169 = call "Actualizar_Interfaz.vi"("Enum"=Acciones_UI."Desactivar", "Controls"=w450) -> ()  [unwired: 8 in, 2 out]
        n170 = Build Array(w434) -> (w459:refnum<vi>[])
        n171 = call "Actualizar_Interfaz.vi"("Enum"=Acciones_UI."Activar", "Controls"=w459) -> ("Controls 2"=w441:refnum<vi>[])  [unwired: 8 in, 1 out]
        n172 = call "Actualizar_Interfaz.vi"("Enum"=Acciones_UI."Reiniciar default", "Controls"=w441) -> ()  [unwired: 8 in, 2 out]
        n173 = Select(t=ESTADOS."Salir" ("Enum"), s=w443, f=ESTADOS."Ping_Arduino") -> (s? t:f=w444:T2)
      }
      frame "Cabezal Posicion Inicio" {
        n174 = disable-structure shown="Disabled" {
          disable-tunnel: w467 -> [w479 _]
          disable-tunnel: [w475 _] -> w466
          disable-tunnel: w465 -> [w473 _]
          disable-tunnel: w464 -> [w472 _]
          disable-tunnel: [w469 _] -> w463
          frame Disabled {
            # "ENVIO COMANDO PARA POSICION INICIO\nEL ROBOT SE EMPIEZA A MOVER A POSICION\nINICIO"
            # "LEO ESTADO EN ARDUINO"
            n175 = call "Ack_estado_Arduino.vi"("error in (no error)"=w479, "Enum"=Estados_arduino."4", "VISA resource name"=w473) -> ("error out"=w478:errorcluster)  [unwired: 6 in, 2 out]
            n176 = call "Enviar_comando.vi"("error in (no error)"=w478, "Enum"=Comandos."I", "VISA resource name"=w473) -> ("error out"=w470:errorcluster)  [unwired: 6 in, 2 out]
            n177 = Unbundle By Name(w472) -> ("MENSAJES AL USUARIO"=w471:refnum<vi>)
            n178 = property class="Str"(reference=w471, error in=w470, "Text.Text"="CABEZAL YENDO A POSICION DE INICIO") -> (error out=w469:errorcluster)  [unwired: 1 out]
            n179 = Select(t=ESTADOS."Salir", s=w469, f=ESTADOS."Terminaste posicion inicio?" ("Enum")) -> (s? t:f=w475:T2)
          }
          frame Enabled {
          }
        }
      }
      frame "Terminaste posicion inicio?" {
        n180 = disable-structure shown="Disabled" {
          disable-tunnel: [w506 _] -> w486
          disable-tunnel: w485 -> [w505 _]
          disable-tunnel: w484 -> [w493 _]
          disable-tunnel: w483 -> [w492 _]
          disable-tunnel: [w491 _] -> w482
          frame Disabled {
            # "LEO ESTADO EN ARDUINO"
            # "ESPERAR A QUE SE VAYA\nA POSICION INICIO Y NOS ENVIE EL COMANDO\n\"FI\""
            # "ESPERO COMANDO POSICION INICIO\nFINALIZADA"
            n181 = call "Ack_estado_Arduino.vi"("error in (no error)"=w493, "Enum"=Estados_arduino."5", "VISA resource name"=w492) -> ("error out"=w507:errorcluster)  [unwired: 6 in, 2 out]
            n182 = case shown="No Error" w507 {
              selector: w507 -> [w513 w522]
              tunnel: [w515 w522] -> w509
              tunnel: w492 -> [w514 _]
              frame No Error {
                n183 = while {
                  tunnel: [w521] -> w515
                  tunnel: w514 -> [w517]
                  tunnel: w513 -> [w516]
                  stop <- w518 stop-if-true
                  # "POLLING"
                  n184 = property class="Instr"(reference=w517, error in=w516) -> (error out=w521:errorcluster, "Serial Settings:Number of Bytes at Serial Port"=w520:u32)  [unwired: 1 out]
                  n185 = Equal?(x=w520, y=u32 2) -> (x = y?=w518:bool)
                }
              }
              frame Error {
              }
            }
            n186 = call "Ack_comando_arduino.vi"("error in (no error)"=w509, 10:Comandos."FI", "VISA resource name"=w492) -> ("error IO"=w490:errorcluster)  [unwired: 6 in, 2 out]
            n187 = Unbundle By Name(w505) -> ("Retroc"=w504:refnum<vi>, "Home"=w503:refnum<vi>, "Izq"=w502:refnum<vi>, "Der"=w501:refnum<vi>, "Stop Program"=w500:refnum<vi>, "Avanzar"=w499:refnum<vi>, "Bajar Z"=w498:refnum<vi>, "Distancia"=w497:refnum<vi>, "Subir Z"=w496:refnum<vi>, "MENSAJES AL USUARIO"=w489:refnum<vi>)
            n188 = property class="Str"(reference=w489, error in=w490, "Text.Text"="CABEZAL EN POSICION DE INICIO") -> (error out=w487:errorcluster)  [unwired: 1 out]
            n189 = Build Array(w504, w503, w502, w501, w500, w499, w498, w497, w496) -> (w495:refnum<vi>[])
            n190 = call "Actualizar_Interfaz.vi"("error in (no error)"=w487, "Enum"=Acciones_UI."Activar", "Controls"=w495) -> ("error out"=w491:errorcluster)  [unwired: 7 in, 1 out]
            n191 = Select(t=ESTADOS."Salir" ("Enum"), s=w491, f=ESTADOS."Check Button") -> (s? t:f=w506:T2)
          }
          frame Enabled {
          }
        }
      }
      frame "Ping_Arduino" {
        n192 = VISA Write(VISA resource name=w524, write buffer="Q?", error in (no error)=w533) -> (return count=w536:u32, error out=w535:errorcluster)  [unwired: 1 out]
        n193 = VISA Read(VISA resource name=w524, byte count=w536, error in (no error)=w535) -> (read buffer=w531:string, error out=w530:errorcluster)  [unwired: 2 out]
        n194 = Equal?(x=w531, y="R!") -> (x = y?=w532:bool)
        n195 = case shown="True" w532 {
          tunnel: w531 -> [w544 _]
          tunnel: w530 -> [w542 w559]
          tunnel: [w541 w559] -> w523
          tunnel: w526 -> [w539 w557]
          frame False {
            n196 = Unbundle By Name(w539) -> ("MENSAJES AL USUARIO"=w538:refnum<vi>)
            n197 = xnode "Error Ring"("parameter 0"=w544) -> ("error out"=w543:errorcluster)
            n198 = property class="Str"(reference=w538, "Text.Text"="LA COMUNICACION CON ARDUINO HA FALLADO") -> ()  [unwired: 1 in, 2 out]
            n199 = Merge Errors(w543, w542) -> (w541:errorcluster)
          }
          frame True {
            n200 = Unbundle By Name(w557) -> ("Comenzar mov"=w555:refnum<vi>, "MENSAJES AL USUARIO"=w556:refnum<vi>, "Stop Program"=w552:refnum<vi>)
            n201 = Build Array(w555, w552) -> (w554:refnum<vi>[])
            n202 = call "Actualizar_Interfaz.vi"("Enum"=Acciones_UI."Activar", "Controls"=w554) -> ()  [unwired: 8 in, 2 out]
            n203 = property class="Str"(reference=w556, "Text.Text"="COMUNICACION ESTABLECIDA") -> ()  [unwired: 1 in, 2 out]
          }
        }
        n204 = Select(t=ESTADOS."Salir" ("Enum"), s=w523, f=ESTADOS."Check Button") -> (s? t:f=w527:T2)
      }
    }
    "ESTADO FSM" <- w27
    "MOVIMIENTO SOLICITADO" <- w31
    n205 = Equal?(x=w27, y=ESTADOS."Salir") -> (x = y?=w24:bool)
    n206 = Or(x=w25, y=w24) -> (x .or. y?=w28:bool)
  }
  n207 = control-ref of="Movimiento ejecutado?"() -> ()  [unwired: 1 out]
  n208 = VISA Close(VISA resource name=w11, error in (no error)=w10) -> ()  [unwired: 1 out]
